vi "Data Insert.vi"() -> ()   [LabVIEW 2019]
uses:
  data.ctl
  <vilib>/addons/database/Connection.llb/DB Tools Open Connec (String).vi
  <vilib>/addons/database/NI_Database_API.lvlib
panel:
  in  "Data":T1
  in  "table":string
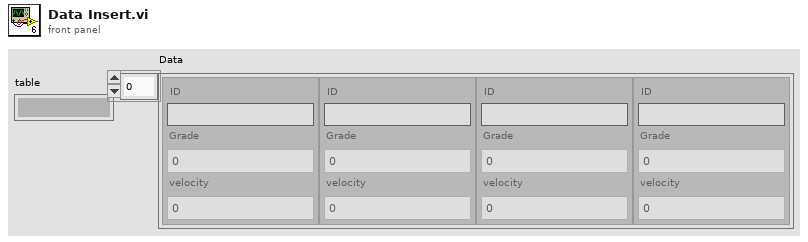
[diagram p1: front panel]
types:
  T1 = typedef "data.ctl" = cluster{"ID":string, "Grade":dbl, "velocity":dbl}[]
  T2 = typedef "NI_Database_API.lvlib/Conn ObjectReference.ctl" = refnum<k1>
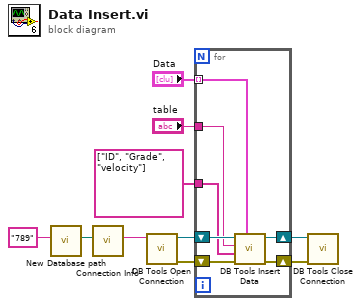
[diagram p0: block diagram]
diagram:
  n1 = call "New Database path.vi"("Database Name"="789") -> ("Database path"=w10:path)  [unwired: 10 in]
  n2 = call "Connection Info.vi"("路径"=w10) -> ("Connection Info"=w4:string)  [unwired: 10 in]
  n3 = call-poly <vilib>:"DB Tools Open Connection.vi"("connection information"=w4) -> ("error out"=w5:errorcluster, "connection reference"=w8:T2)  [unwired: 7 in]
  n4 = for {
    tunnel: "table" -> [w13]
    tunnel: string[] ["ID", "Grade", "velocity"] ("columns") -> [w12]
    tunnel: "Data" -> [w11] mode=indexing
    shift-right: [w16] -> w7
    shift-left: w8 -> [w17]
    shift-right: [w15] -> w6
    shift-left: w5 -> [w14]
    n5 = call <vilib>:"DB Tools Insert Data.vi"("data"=w11, "error in (no error)"=w14, "columns"=w12, "table"=w13, "connection reference"=w17) -> ("error out"=w15:errorcluster, "connection reference out"=w16:T2)  [unwired: 5 in]
  }
  n6 = call <vilib>:"DB Tools Close Connection.vi"("error in (no error)"=w6, "connection reference"=w7) -> ()  [unwired: 5 in, 1 out]
